vi "Start Analog Output.vi"(8 "error in (no error)":errorcluster) -> (0 "error out":errorcluster, 3 "AO Task ID's Out":u32[](array[numeric]))   [LabVIEW 2009]
uses:
  Acquisition Settings.vi
  <vilib>/Daq/ao.llb/AO Write (scaled array).vi
panel:
  out "Output Data":dbl[][](graph)
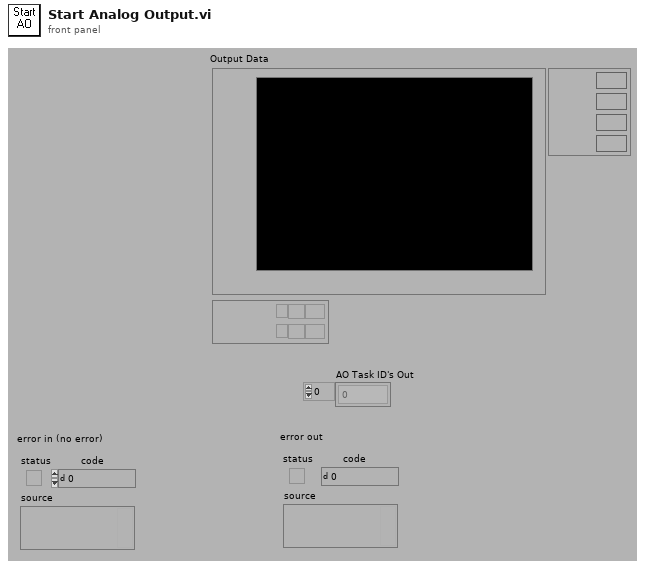
[diagram p1: front panel]
types:
  T1 = cluster{"device":i16, "channel":tag, "buffer size":i32, "Signal Description":cluster{"Name":string, "signal type":enum16{"Sine Wave", "Square Wave", "Sawtooth", "Triangle Wave"}, "period":dbl, "amplitude":dbl, "phase (0 deg)":dbl, "offset (0.0)":dbl, "resting voltage":dbl, "% duty cycle":dbl}[], "clock source (internal:1)":u16, "Clock Line Number":i16}[]
  T2 = cluster{"Name":string, "signal type":enum16{"Sine Wave", "Square Wave", "Sawtooth", "Triangle Wave"}, "period":dbl, "amplitude":dbl, "phase (0 deg)":dbl, "offset (0.0)":dbl, "resting voltage":dbl, "% duty cycle":dbl}[]
  T3 = enum16{"Sine Wave", "Square Wave", "Sawtooth", "Triangle Wave"}
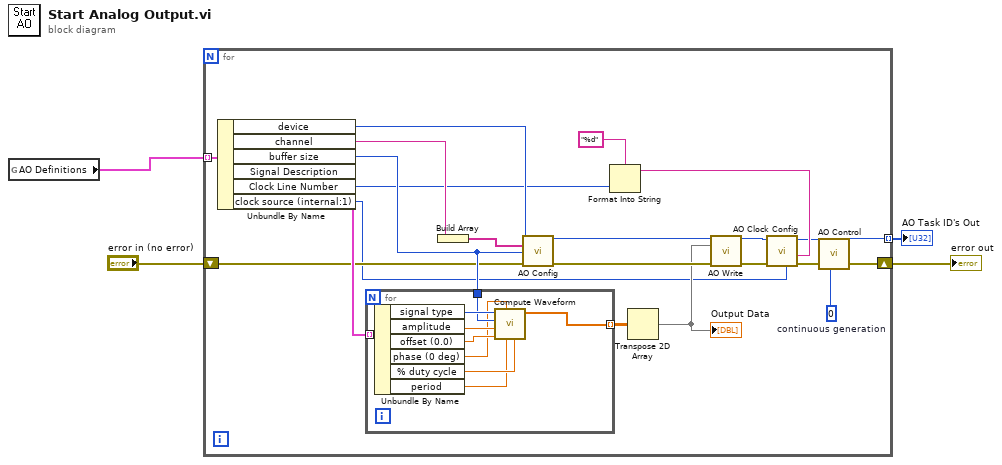
[diagram p0: block diagram]
diagram:
  n1 = global read "Acquisition Settings.vi" "AO Definitions"() -> (w1:T1)
  n2 = for {
    tunnel: w1 -> [w23] mode=indexing
    tunnel: [w7] -> w4 mode=indexing
    shift-right: [w6] -> w2
    shift-left: "error in (no error)" -> [w17]
    w14 = 0  # continuous generation
    n3 = Unbundle By Name(w23) -> ("device"=w24:i16, "channel"=w22:tag, "buffer size"=w20:i32, "Signal Description"=w21:T2, "Clock Line Number"=w12:i16, "clock source (internal:1)"=w5:u16)
    n4 = for {
      tunnel: w21 -> [w35] mode=indexing
      tunnel: w20 -> [w32]
      tunnel: [w29] -> w19 mode=indexing
      n5 = Unbundle By Name(w35) -> ("signal type"=w34:T3, "amplitude"=w33:dbl, "offset (0.0)"=w31:dbl, "phase (0 deg)"=w30:dbl, "% duty cycle"=w28:dbl, "period"=w27:dbl)
      n6 = call "Compute Waveform.vi"("% duty cycle\n(square wave only, 50)"=w28, "Period"=w27, "phase (0 deg)"=w30, "offset (0.0)"=w31, "amplitude (1.0)"=w33, "number of points (1000)"=w32, "signal type (0:sine)"=w34) -> ("output waveform"=w29:dbl[])  [unwired: 4 in]
    }
    n7 = Build Array(w22) -> (w25:tag[])
    n8 = call <vilib>:"AO Config.vi"("device (1)"=w24, "channels (0)"=w25, "buffer size (1000 updates)"=w20, "error in (no error)"=w17) -> ("taskID"=w13:u32, "error out"=w26:errorcluster)  [unwired: 9 in, 1 out]
    n9 = Format Into String(format string="%d" ("Format String"), w12) -> (resulting string=w10:string)  [unwired: 2 in, 1 out]
    n10 = Transpose 2D Array(2D array=w19) -> (transposed array=w18:dbl[][])
    "Output Data" <- w18
    n11 = call-poly <vilib>:"AO Write.vi"("taskID in"=w13, "scaled data"=w18, "error in (no error)"=w26) -> ("taskID out"=w16:u32, "error out"=w15:errorcluster)  [unwired: 8 in, 3 out]
    n12 = call <vilib>:"AO Clock Config.vi"("clock source specification"=w10, "clock source (0: no change)"=w5, "error in (no error)"=w15, "task ID"=w16) -> ("error out"=w8:errorcluster, "task ID out"=w9:u32)  [unwired: 5 in, 1 out]
    n13 = call <vilib>:"AO Control.vi"("iterations (0: infinite)"=w14, "error in (no error)"=w8, "task ID"=w9) -> ("error out"=w6:errorcluster, "task ID out"=w7:u32)  [unwired: 7 in]
  }
  "AO Task ID's Out" <- w4
  "error out" <- w2
